vi "DUAL GAUGE-RW Sensor Control.vi"(0 "Referenz in":refnum<visa-resource-name>, 1 "Controlling source deactivation":i32(ring)=2 items=["no control", "automatic deactivation", "manual deactivation (default)", "external deactivation", "self control"], 2 "Controlling source activation":i32(ring)=2 items=["no control", "automatic activation", "manual activation (default)", "external activation", "hot start"], 3 "ON threshold":dbl=0.001 min=0.0 max=41000.0 format="%.2e", 4 "OFF threshold":dbl=0.001 min=0.0 max=41000.0 format="%.2e", 5 "Fehler (Eingang)":errorcluster, 6 "Gauge Nr.":i32(ring) items=["CH 1", "CH 2"], 8 "W/R":bool) -> (14 "Referenz out":refnum<visa-resource-name>, 15 "Controlling source deactivation out":i32(ring)=2 items=["no control", "automatic deactivation", "manual deactivation (default)", "external deactivation", "self control"], 16 "Controlling source activation out":i32(ring)=2 items=["no control", "automatic activation", "manual activation (default)", "external activation", "hot start"], 17 "Get ON threshold":dbl min=0.0 max=41000.0 format="%.2e", 18 "Get OFF threshold":dbl min=0.0 max=41000.0 format="%.2e", 19 "Cluster (Ausgang)":errorcluster)   [LabVIEW 2013, in "Dual Gauge.lvlib"]
uses:
  Dual Gauge.lvlib
panel:
  # "mbar"
  # "mbar"
  # "mbar"
  # "mbar"
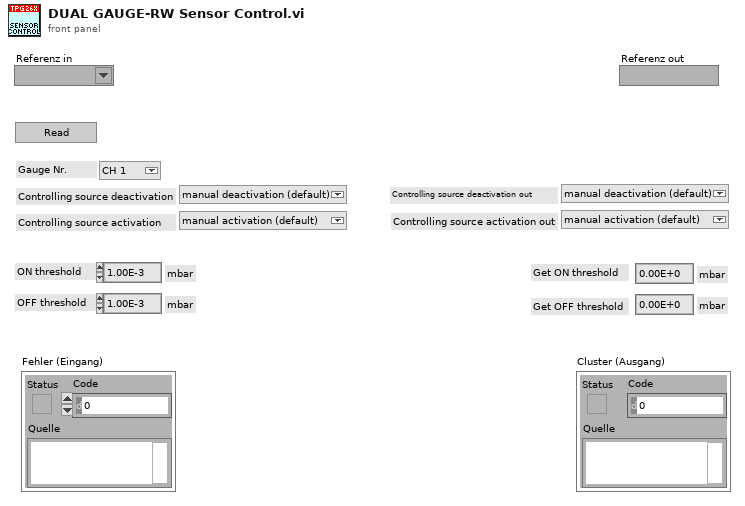
[diagram p1: front panel]
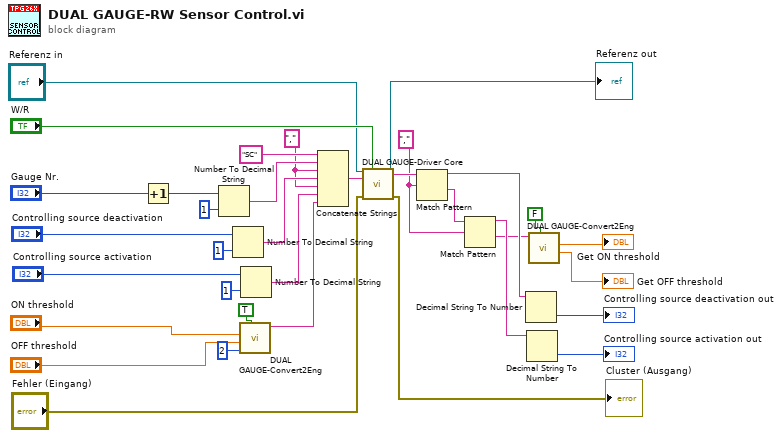
[diagram p0: block diagram]
diagram:
  w7 = "," ("Command")
  w14 = "," ("Command")
  n1 = Increment(x="Gauge Nr.") -> (x+1=w29:i32)
  n2 = Number To Decimal String(number=w29, width (-)=i16 1) -> (decimal integer string=w17:string)
  n3 = Number To Decimal String(number="Controlling source deactivation", width (-)=i16 1) -> (decimal integer string=w15:string)
  n4 = call "DUAL GAUGE-Convert2Eng.vi"("W/R [W: Int in; Str out ]"=TRUE, "Kommastellen"=u8 2, "Eng2 in"="OFF threshold", "Eng1 in"="ON threshold") -> ("String out"=w12:string)  [unwired: 5 in, 2 out]
  n5 = Number To Decimal String(number="Controlling source activation", width (-)=i16 1) -> (decimal integer string=w13:string)
  n6 = Concatenate Strings("SC" ("Command"), w17, w14, w15, w14, w13, w12) -> (w5:string)
  n7 = call "DUAL GAUGE-Driver Core.vi"("Referenz in"="Referenz in", "Write/Read"="W/R", "Command"=w5, "Fehler (Eingang)"="Fehler (Eingang)") -> ("Referenz out"=→"Referenz out":refnum<visa-resource-name>, "String Out"=w11:string, "Cluster (Ausgang)"=→"Cluster (Ausgang)":errorcluster)  [unwired: 9 in]
  n8 = Match Pattern(string=w11, regular expression=w7) -> (before substring=w10:string, after substring=w6:string)  [unwired: 1 in, 2 out]
  n9 = Match Pattern(string=w6, regular expression=w7) -> (before substring=w9:string, after substring=w8:string)  [unwired: 1 in, 2 out]
  n10 = Decimal String To Number(string=w10) -> (number=→"Controlling source deactivation out":i32)  [unwired: 2 in, 1 out]
  n11 = Decimal String To Number(string=w9) -> (number=→"Controlling source activation out":i32)  [unwired: 2 in, 1 out]
  n12 = call "DUAL GAUGE-Convert2Eng.vi"("W/R [W: Int in; Str out ]"=FALSE, "String in"=w8) -> ("Eng2 out"=→"Get OFF threshold":dbl, "Eng1 out"=→"Get ON threshold":dbl)  [unwired: 7 in, 1 out]
